vi "Draw Trajectory.vi"(0 "Picture in":refnum<vi>, 1 "Robot Index":i32, 5 "Trajectory Data":T3, 7 "time":dbl, 9 "new picture in":picture, 10 "MEGA?":bool, 11 "Hide Path":bool, 12 "MEGA traj":T2 {"?"."Limits"."StoopidFast (fps)" min=0.0; "?"."Limits"."Jerk (fps^3)" min=0.0 step=1.0; "?"."Limits"."Accel (fps^2)" min=0.0; "?"."Limits"."Velocity (fps)" min=0.0; "?"."Overrides"."Angle Override" step=5.0; "?"."Overrides"."Velocity Override" step=5.0; "?"."Overrides"."Angular Override" step=5.0; "?"."Angular Limits"."Jerk (deg/s^3)" min=0.0 step=1.0; "?"."Angular Limits"."Accel (deg/s^2)" min=0.0; "?"."Angular Limits"."Velocity (deg/s)" min=0.0}, 13 "color(black)":u32(colorbox)=6618880) -> (3 "Path Points MEGA":cluster{"x":dbl, "y":dbl}[][](array[cluster]), 4 "new picture":picture, 6 "Output Point":T12, 14 "Output Point MEGA":T1(array[cluster]), 15 "Path Points":cluster{"x":dbl, "y":dbl}[](array[cluster]))   [LabVIEW 2025]
uses:
  Types/Trajectory Data.ctl
  Types/Segment Type.ctl
  FileIO/MEGA traj.ctl
  Types/Single Cmd Info.ctl
  <vilib>/picture/picture.llb/imagedata.ctl
  Types/Limits.ctl
  Types/Overrides.ctl
  Types/Angluar Limits.ctl
  Types/Drive Type.ctl
  Types/Path Type.ctl
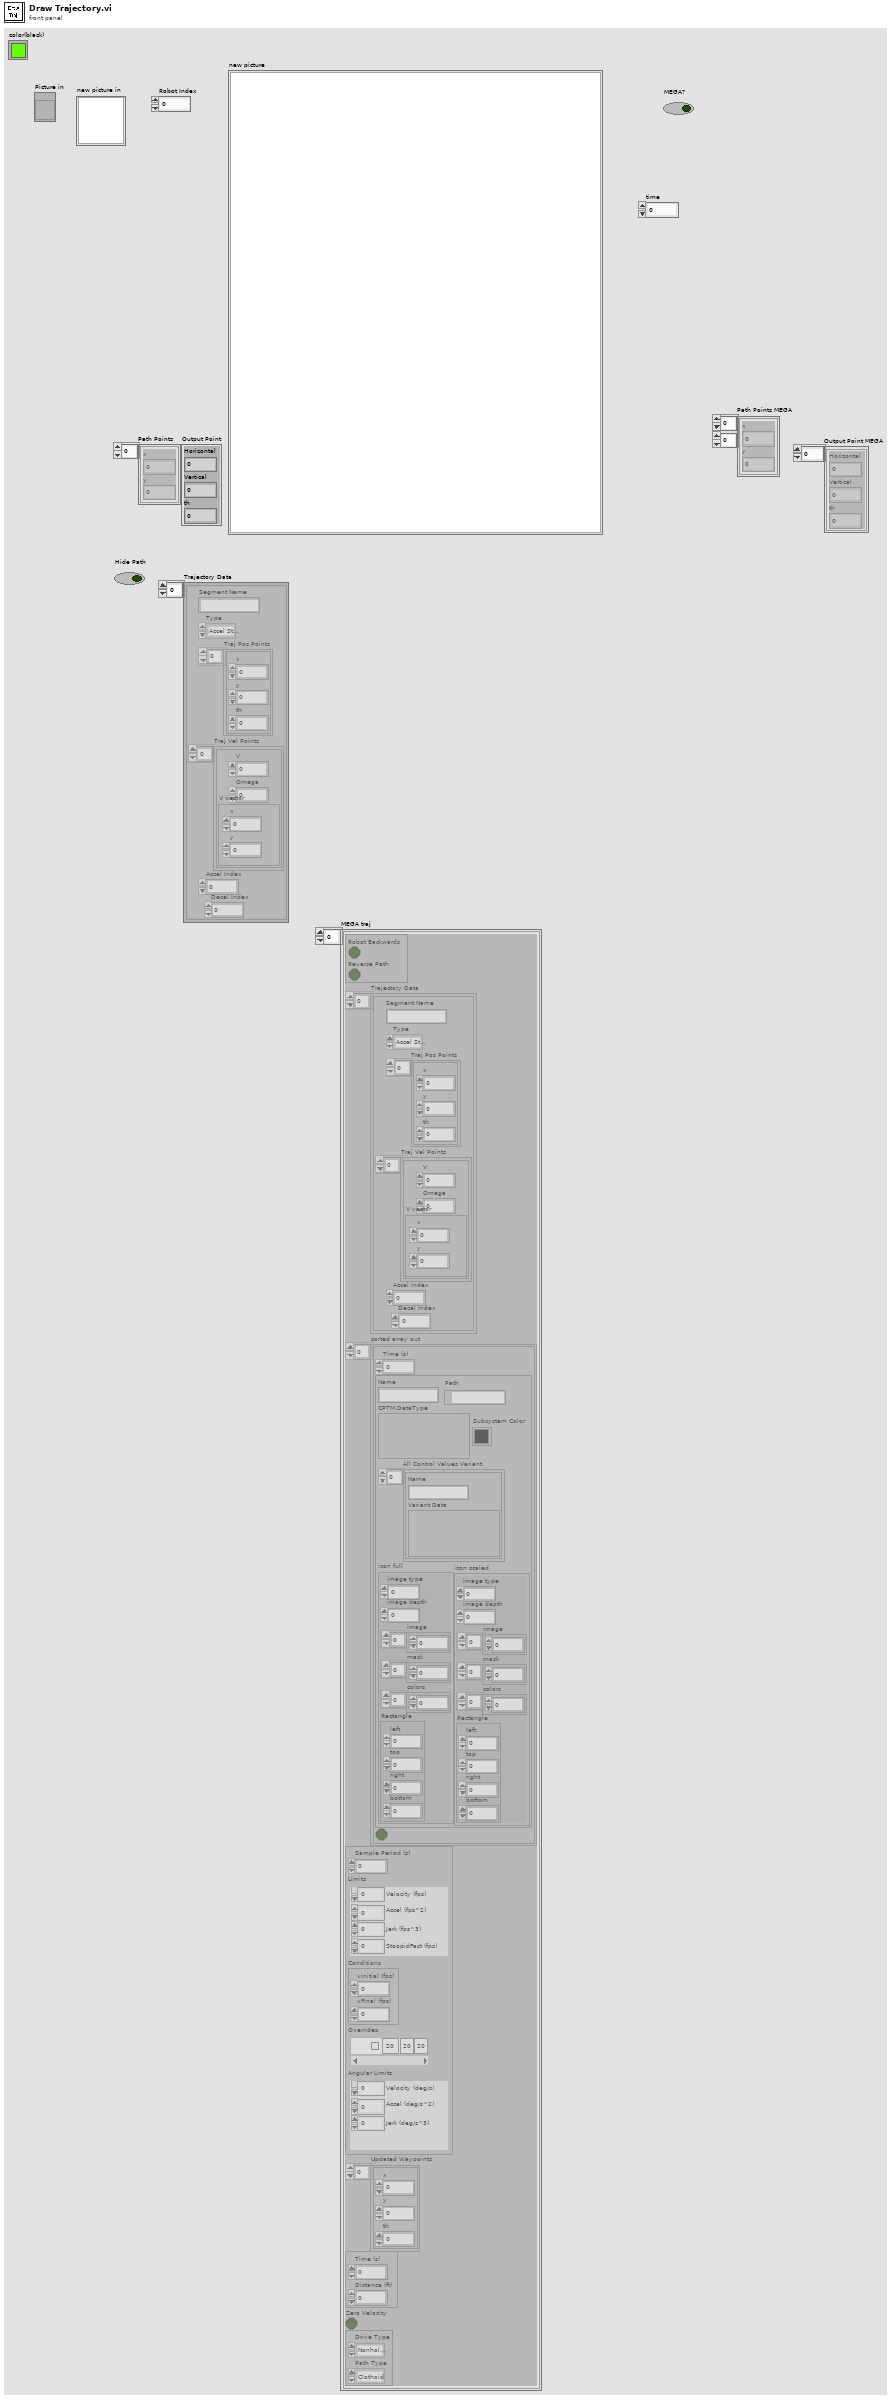
[diagram p1: front panel]
types:
  T1 = cluster{"Horizontal":dbl, "Vertical":dbl, "th":dbl}[]
  T2 = typedef "MEGA traj.ctl" = cluster{cluster{"Robot Backwards":bool, "Reverse Path":bool}, "Trajectory Data":T3, "sorted array out":cluster{"Time (s)":dbl, T5, bool}[], cluster{"Sample Period (s)":dbl, "Limits":T7, "Conditions":cluster{"vInitial (fps)":dbl, "vFinal (fps)":dbl}, "Overrides":T8, "Angular Limits":T9}, "Updated Waypoints":cluster{"x":dbl, "y":dbl, "th":dbl}[], cluster{"Time (s)":dbl, "Distance (ft)":dbl}, "Zero Velocity":bool, cluster{"Drive Type":T10, "Path Type":T11}}[]
  T3 = typedef "Trajectory Data.ctl" = cluster{"Segment Name":string, "Type":T4, "Traj Pos Points":cluster{"x":dbl, "y":dbl, "th":dbl}[], "Traj Vel Points":cluster{"V":dbl, "Omega":dbl, "V vector":cluster{"y":dbl, "x":dbl}}[], "Accel Index":i32, "Decel Index":i32}[]
  T4 = typedef "Segment Type.ctl" = enum16{"Accel Straight", "Const Straight", "Blend", "Circle", "Bezier"}
  T5 = typedef "Single Cmd Info.ctl" = cluster{"Name":string, "CPTM.DataType":variant, "All Control Values Variant":cluster{"Name":string, "Variant Data":variant}[], "icon full":T6, "icon scaled":T6, "Path":path, "Subsystem Color":u32}
  T6 = typedef "imagedata.ctl" = cluster{"image type":i32, "image depth":i32, "image":u8[], "mask":u8[], "colors":u32[], "Rectangle":cluster{"left":i16, "top":i16, "right":i16, "bottom":i16}}
  T7 = typedef "Limits.ctl" = cluster{"Velocity (fps)":dbl, "Accel (fps^2)":dbl, "Jerk (fps^3)":dbl, "StoopidFast (fps)":dbl}
  T8 = typedef "Overrides.ctl" = cluster{"Count":string, "Angular Override":dbl, "Enabled?":bool, "Velocity Override":dbl, "Angle Override":dbl}[]
  T9 = typedef "Angluar Limits.ctl" = cluster{"Velocity (deg/s)":dbl, "Accel (deg/s^2)":dbl, "Jerk (deg/s^3)":dbl}
  T10 = typedef "Drive Type.ctl" = enum16{"Nonholonomic", "Holonomic"}
  T11 = typedef "Path Type.ctl" = enum16{"Clothoid", "Bezier"}
  T12 = cluster{"Horizontal":dbl, "Vertical":dbl, "th":dbl}
  T13 = cluster{"Width":u16, "Style":enum32{"Solid", "Dash", "Dot", "DashDot", "DashDotDot"}}
  T14 = typedef "LVPositionTypeDef.ctl" = cluster{"Left":i32, "Top":i32}
  T15 = typedef "LVBoundsTypeDef.ctl" = cluster{"Width":u32, "Height":u32}
  T16 = cluster{"V":dbl, "Omega":dbl, "V vector":cluster{"y":dbl, "x":dbl}}[]
  T17 = cluster{cluster{"Robot Backwards":bool, "Reverse Path":bool}, "Trajectory Data":T3, "sorted array out":cluster{"Time (s)":dbl, T5, bool}[], cluster{"Sample Period (s)":dbl, "Limits":T7, "Conditions":cluster{"vInitial (fps)":dbl, "vFinal (fps)":dbl}, "Overrides":T8, "Angular Limits":T9}, "Updated Waypoints":cluster{"x":dbl, "y":dbl, "th":dbl}[], cluster{"Time (s)":dbl, "Distance (ft)":dbl}, "Zero Velocity":bool, cluster{"Drive Type":T10, "Path Type":T11}}
  T18 = cluster{"Robot Backwards":bool, "Reverse Path":bool}
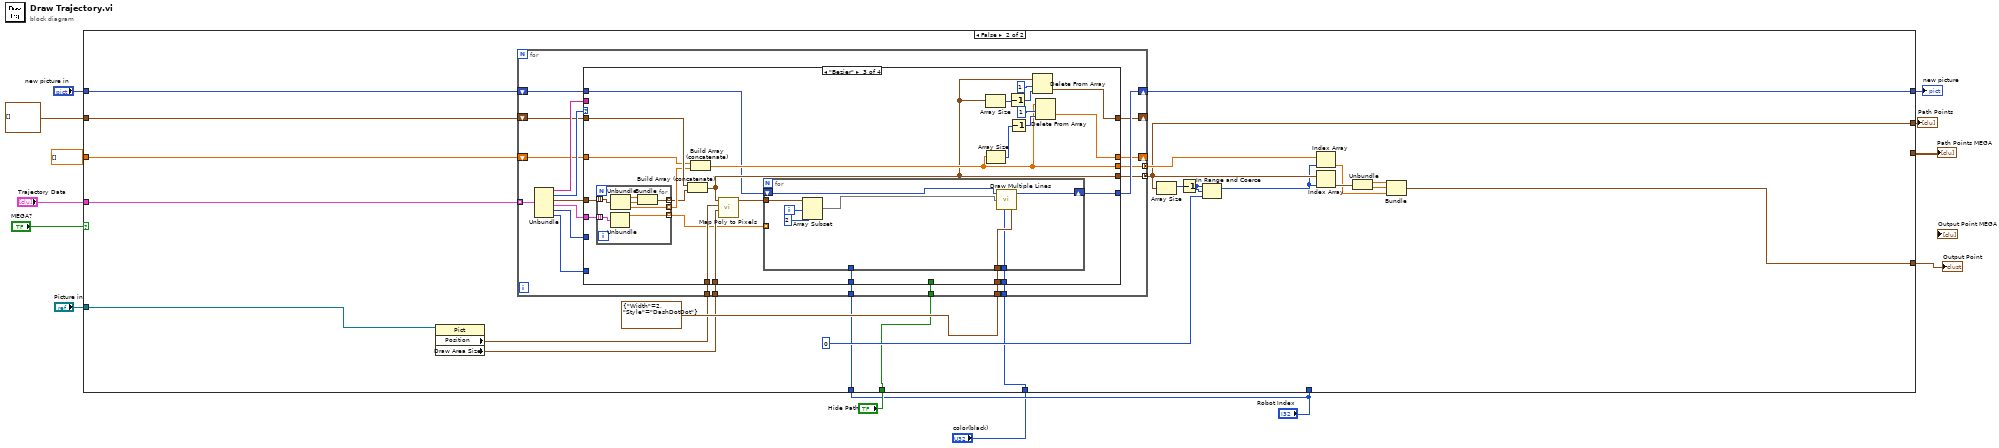
[diagram p0: block diagram]
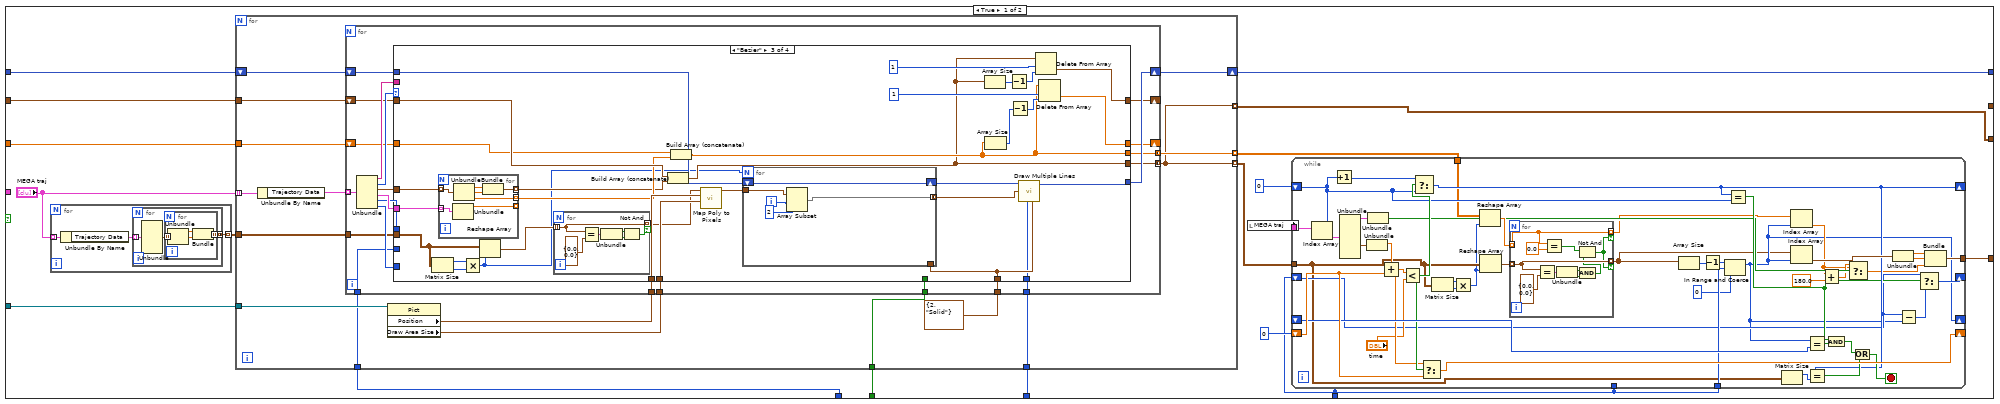
[diagram p2: hidden frame]
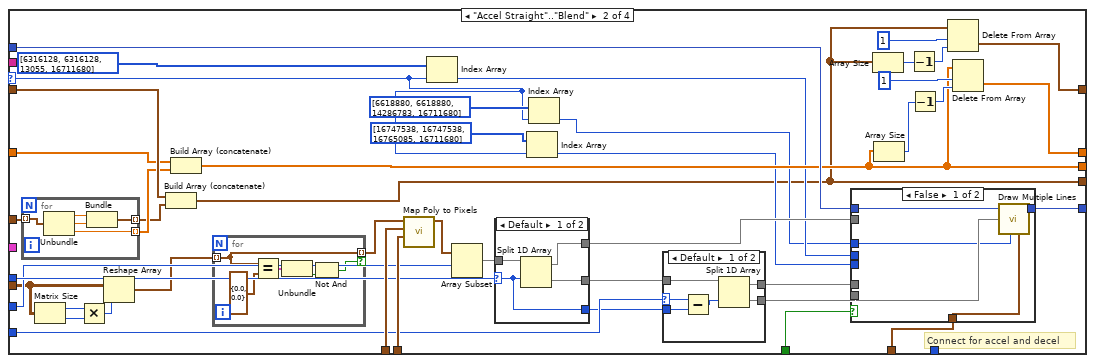
[diagram p4: hidden frame]
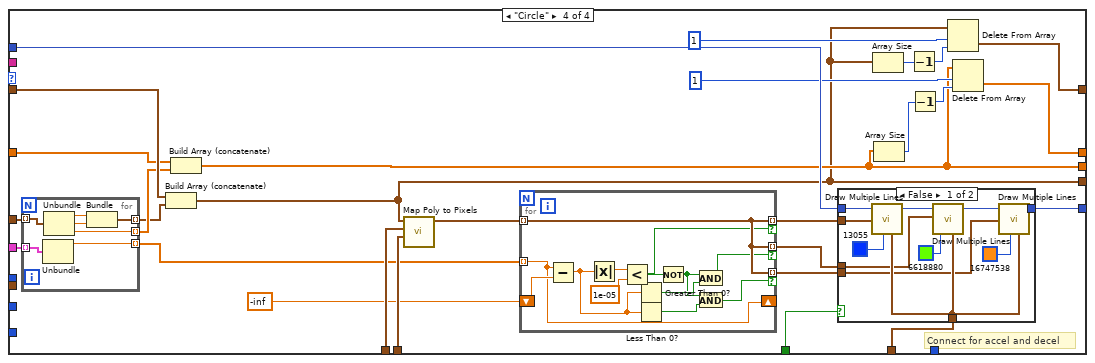
[diagram p8: hidden frame]
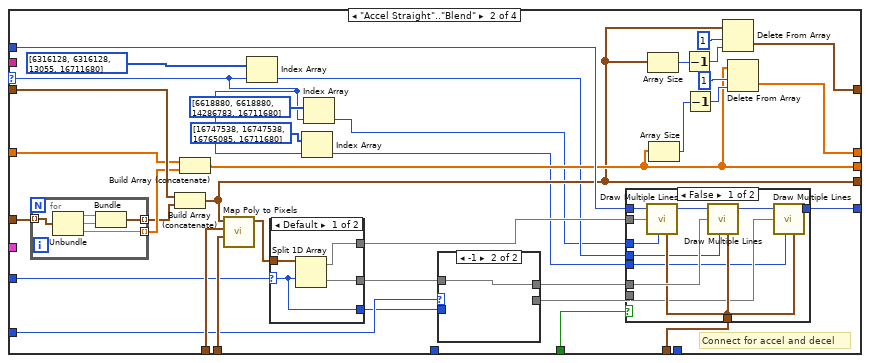
[diagram p11: hidden frame]
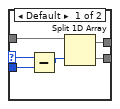
[diagram p13: hidden frame]
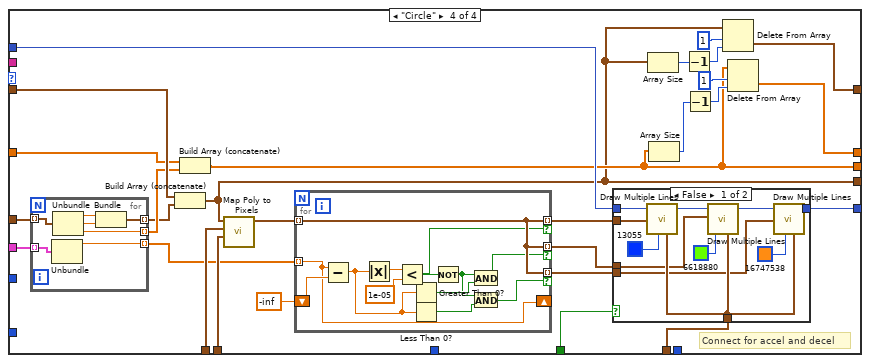
[diagram p15: hidden frame]
diagram:
  n1 = case shown="False" "MEGA?" {
    tunnel: "Picture in" -> [w31 w342]
    tunnel: "new picture in" -> [w30 w341]
    tunnel: [w29 w337] -> w11
    tunnel: [_ w331] -> w10
    tunnel: cluster{"x":dbl, "y":dbl}[] [] -> [w28 w327]
    tunnel: dbl[] [] -> [w27 w326]
    tunnel: "Trajectory Data" -> [_ w325]
    tunnel: "Hide Path" -> [w26 w324]
    tunnel: [w19 _] -> w4
    tunnel: "Robot Index" -> [w18 _]
    tunnel: [w23 w323] -> w3
    tunnel: "Robot Index" -> [w17 w322]
    tunnel: "color(black)" -> [w14 w321]
    frame True {
      n2 = for {
        tunnel: "MEGA traj" -> [w34] mode=indexing
        tunnel: [w32] -> w15 mode=indexing
        n3 = Unbundle By Name(w34) -> ("Trajectory Data"=w33:T3)
        n4 = for {
          tunnel: w33 -> [w37] mode=indexing
          tunnel: [w35] -> w32 mode=concatenating
          n5 = Unbundle(w37) -> ("Traj Pos Points"=w36:cluster{"x":dbl, "y":dbl, "th":dbl}[])  [unwired: 5 out]
          n6 = for {
            tunnel: w36 -> [w39] mode=indexing
            tunnel: [w38] -> w35 mode=indexing
            n7 = Unbundle(w39) -> ("x"=w41:dbl, "y"=w40:dbl)  [unwired: 1 out]
            n8 = Bundle("x"=w41, "y"=w40) -> (w38:cluster{"x":dbl, "y":dbl})  [unwired: 1 in]
          }
        }
      }
      n9 = for {
        tunnel: w31 -> [w113]
        tunnel: [w102] -> w19 mode=indexing
        tunnel: w28 -> [w107]
        tunnel: w27 -> [w106]
        shift-right: [w108] -> w29
        shift-left: w30 -> [w112]
        tunnel: w26 -> [w105]
        tunnel: "MEGA traj" -> [w100] mode=indexing
        tunnel: [w103] -> w20 mode=indexing
        tunnel: [w102] -> w21 mode=indexing
        tunnel: w17 -> [w101]
        tunnel: w15 -> [w99]
        tunnel: w14 -> [w98]
        n10 = Unbundle By Name(w100) -> ("Trajectory Data"=w104:T3)
        n11 = property on="Property Node" class="Pict"(reference=w113) -> ("Position"=w109:T14, "Draw Area Size"=w110:T15)  [unwired: 1 in, 2 out]
        n12 = for {
          tunnel: w104 -> [w135] mode=indexing
          shift-right: [w129] -> w108
          shift-left: w112 -> [w128]
          tunnel: T13 {"Width"=2, "Style"=enum."Solid"} ("pen") -> [w132]
          tunnel: w110 -> [w131]
          tunnel: w109 -> [w130]
          tunnel: [w126] -> w102 mode=concatenating
          tunnel: [w125] -> w103 mode=concatenating
          shift-right: [w124] -> _
          shift-left: w107 -> [w123]
          shift-right: [w122] -> _
          shift-left: w106 -> [w121]
          tunnel: w105 -> [w119]
          tunnel: w101 -> [w116]
          tunnel: w99 -> [w115]
          tunnel: w98 -> [w114]
          n13 = Unbundle(w135) -> ("Segment Name"=w134:string, "Type"=w127:T4, "Traj Pos Points"=w117:cluster{"x":dbl, "y":dbl, "th":dbl}[], "Traj Vel Points"=w133:T16, "Accel Index"=w118:i32, "Decel Index"=w120:i32)
          n14 = case shown="\"Bezier\"" w127 {
            selector: w127 -> [_ w152 _ _]
            tunnel: w134 -> [_ _ _ _]
            tunnel: w117 -> [_ w182 w242 w288]
            tunnel: w133 -> [_ _ w225 w267]
            tunnel: w132 -> [_ w161 w215 w271]
            tunnel: w131 -> [_ w181 w241 w287]
            tunnel: w130 -> [_ w179 w240 w285]
            tunnel: [w138 w162 w214 w272] -> w129
            tunnel: w128 -> [w138 w180 w224 w286]
            tunnel: [_ w146 w226 w269] -> w126
            tunnel: [_ w168 w230 w275] -> w125
            tunnel: w118 -> [_ w165 _ _]
            tunnel: [w137 w173 w235 w280] -> w124
            tunnel: w123 -> [w137 w176 w238 w283]
            tunnel: [w136 w169 w231 w276] -> w122
            tunnel: w121 -> [w136 w166 w228 w273]
            tunnel: w120 -> [_ w164 _ _]
            tunnel: w119 -> [_ w149 _ w268]
            tunnel: w116 -> [_ w145 _ _]
            tunnel: w115 -> [_ w144 w221 _]
            tunnel: w114 -> [_ _ w212 _]
            frame Default {
            }
            frame "Accel Straight".."Blend" {
              # "Connect for accel and decel"
              n15 = for {
                tunnel: w182 -> [w211] mode=indexing
                tunnel: [w210] -> w157 mode=indexing
                tunnel: [w207] -> w167 mode=indexing
                n16 = Unbundle(w211) -> ("x"=w209:dbl, "y"=w208:dbl, "th"=w207:dbl)
                n17 = Bundle("x"=w209, "y"=w208) -> (w210:cluster{"x":dbl, "y":dbl})  [unwired: 1 in]
              }
              n18 = Matrix Size(0:w144) -> (1:w143:i32, 2:w142:i32)
              n19 = Multiply(x=w143, y=w142) -> (x*y=w141:i32)
              n20 = Reshape Array(w144, w141) -> (w140:cluster{"x":dbl, "y":dbl}[])
              n21 = Build Array (concatenate)(w176, w157) -> (w146:cluster{"x":dbl, "y":dbl}[])
              n22 = Build Array (concatenate)(w166, w167) -> (w168:dbl[])
              n23 = for {
                tunnel: w140 -> [w188] mode=indexing
                tunnel: [w188] -> w139 mode=indexing if=w183
                n24 = Equal?(x=w188, y=cluster{"x":dbl, "y":dbl} {"x"=0.0, "y"=0.0}) -> (x = y?=w186:cluster{"x":bool, "y":bool})
                n25 = Unbundle(w186) -> ("x"=w184:bool, "y"=w185:bool)
                n26 = Not And(1:w185, 2:w184) -> (0:w183:bool)
              }
              n27 = call "Map Poly to Pixels.vi"("Draw Area Size"=w181, "Position"=w179, "Coords"=w139) -> ("Coords"=w147:cluster{"Horizontal":dbl, "Vertical":dbl}[])  [unwired: 8 in]
              n28 = Index Array(array=u32[] [6316128, 6316128, 13055, 16711680], index=w152) -> (element=w155:u32)
              n29 = Array Subset(array=w147, index=w145) -> (w148:cluster{"Horizontal":dbl, "Vertical":dbl}[])  [unwired: 1 in]
              n30 = case shown="Default" w165 {
                selector: w165 -> [w202 _]
                tunnel: w148 -> [w205 w206]
                tunnel: [w203 _] -> w156
                tunnel: [w204 w206] -> w159
                tunnel: [w202 _] -> w158
                frame Default {
                  n31 = Split 1D Array(array=w205, index=w202) -> (first subarray=w203:cluster{"Horizontal":dbl, "Vertical":dbl}[], second subarray=w204:cluster{"Horizontal":dbl, "Vertical":dbl}[])
                }
                frame -1 {
                }
              }
              n32 = Index Array(array=u32[] [16747538, 16747538, 16765085, 16711680], index=w152) -> (element=w150:u32)
              n33 = Index Array(array=u32[] [6618880, 6618880, 14286783, 16711680], index=w152) -> (element=w151:u32)
              n34 = case shown="Default" w164 {
                selector: w164 -> [w197 _]
                tunnel: w159 -> [w200 w201]
                tunnel: [w199 w201] -> w163
                tunnel: [w198 _] -> w160
                tunnel: w158 -> [w196 _]
                frame Default {
                  n35 = Subtract(x=w197, y=w196) -> (x-y=w195:i32)
                  n36 = Split 1D Array(array=w200, index=w195) -> (first subarray=w199:cluster{"Horizontal":dbl, "Vertical":dbl}[], second subarray=w198:cluster{"Horizontal":dbl, "Vertical":dbl}[])
                }
                frame -1 {
                }
              }
              n37 = case shown="False" w149 {
                tunnel: w180 -> [w190 w194]
                tunnel: w163 -> [_ _]
                tunnel: [w193 w194] -> w162
                tunnel: w161 -> [w192 _]
                tunnel: w160 -> [w191 _]
                tunnel: w156 -> [_ _]
                tunnel: w155 -> [_ _]
                tunnel: w151 -> [w189 _]
                tunnel: w150 -> [_ _]
                frame False {
                  n38 = call <vilib>:"Draw Multiple Lines.vi"("picture"=w190, "line endpoints"=w191, "color(black)"=w189, "pen"=w192) -> ("new picture"=w193:picture)  [unwired: 5 in]
                }
                frame True {
                }
              }
              n39 = Array Size(array=w146) -> (size(s)=w177:i32)
              n40 = Array Size(array=w168) -> (size(s)=w170:i32)
              n41 = Decrement(x=w177) -> (x-1=w174:i32)
              n42 = Decrement(x=w170) -> (x-1=w172:i32)
              n43 = Delete From Array(array=w146, length=1, index=w174) -> (deleted portion=w173:cluster{"x":dbl, "y":dbl}[])  [unwired: 1 out]
              n44 = Delete From Array(array=w168, length=1, index=w172) -> (deleted portion=w169:dbl[])  [unwired: 1 out]
            }
            frame "Bezier" {
              n45 = Matrix Size(0:w221) -> (1:w220:i32, 2:w223:i32)
              n46 = for {
                tunnel: w242 -> [w260] mode=indexing
                tunnel: [w259] -> w227 mode=indexing
                tunnel: [w256] -> w229 mode=indexing
                tunnel: w225 -> [w255] mode=indexing
                tunnel: [w254] -> _ mode=indexing
                n47 = Unbundle(w255) -> ("V"=w254:dbl)  [unwired: 2 out]
                n48 = Unbundle(w260) -> ("x"=w258:dbl, "y"=w257:dbl, "th"=w256:dbl)
                n49 = Bundle("x"=w258, "y"=w257) -> (w259:cluster{"x":dbl, "y":dbl})  [unwired: 1 in]
              }
              n50 = Multiply(x=w220, y=w223) -> (x*y=w213:i32)
              n51 = Reshape Array(w221, w213) -> (w222:cluster{"x":dbl, "y":dbl}[])
              n52 = for {
                tunnel: w222 -> [w248] mode=indexing
                tunnel: [w248] -> w219 mode=indexing if=w243
                n53 = Equal?(x=w248, y=cluster{"x":dbl, "y":dbl} {"x"=0.0, "y"=0.0}) -> (x = y?=w246:cluster{"x":bool, "y":bool})
                n54 = Unbundle(w246) -> ("x"=w244:bool, "y"=w245:bool)
                n55 = Not And(1:w245, 2:w244) -> (0:w243:bool)
              }
              n56 = Build Array (concatenate)(w238, w227) -> (w226:cluster{"x":dbl, "y":dbl}[])
              n57 = Build Array (concatenate)(w228, w229) -> (w230:dbl[])
              n58 = call "Map Poly to Pixels.vi"("Draw Area Size"=w241, "Position"=w240, "Coords"=w219) -> ("Coords"=w218:cluster{"Horizontal":dbl, "Vertical":dbl}[])  [unwired: 8 in]
              n59 = for {
                N: w213 -> [_]
                tunnel: w215 -> [_]
                shift-right: [w250] -> w217
                shift-left: w224 -> [w250]
                tunnel: w218 -> [w251]
                tunnel: [w249] -> w216 mode=concatenating
                i -> [w253]
                n60 = Array Subset(array=w251, index=w253, length=2) -> (w249:cluster{"Horizontal":dbl, "Vertical":dbl}[])
              }
              n61 = Array Size(array=w226) -> (size(s)=w239:i32)
              n62 = Array Size(array=w230) -> (size(s)=w232:i32)
              n63 = Decrement(x=w239) -> (x-1=w236:i32)
              n64 = Decrement(x=w232) -> (x-1=w234:i32)
              n65 = call <vilib>:"Draw Multiple Lines.vi"("picture"=w217, "line endpoints"=w216, "color(black)"=w212, "pen"=w215) -> ("new picture"=w214:picture)  [unwired: 5 in]
              n66 = Delete From Array(array=w226, length=1, index=w236) -> (deleted portion=w235:cluster{"x":dbl, "y":dbl}[])  [unwired: 1 out]
              n67 = Delete From Array(array=w230, length=1, index=w234) -> (deleted portion=w231:dbl[])  [unwired: 1 out]
            }
            frame "Circle" {
              # "Connect for accel and decel"
              n68 = for {
                tunnel: w288 -> [w319] mode=indexing
                tunnel: [w318] -> w270 mode=indexing
                tunnel: [w315] -> w274 mode=indexing
                tunnel: w267 -> [w314] mode=indexing
                tunnel: [w313] -> w266 mode=indexing
                n69 = Unbundle(w314) -> ("V"=w313:dbl)  [unwired: 2 out]
                n70 = Unbundle(w319) -> ("x"=w317:dbl, "y"=w316:dbl, "th"=w315:dbl)
                n71 = Bundle("x"=w317, "y"=w316) -> (w318:cluster{"x":dbl, "y":dbl})  [unwired: 1 in]
              }
              n72 = Build Array (concatenate)(w283, w270) -> (w269:cluster{"x":dbl, "y":dbl}[])
              n73 = Build Array (concatenate)(w273, w274) -> (w275:dbl[])
              n74 = call "Map Poly to Pixels.vi"("Draw Area Size"=w287, "Position"=w285, "Coords"=w269) -> ("Coords"=w261:cluster{"Horizontal":dbl, "Vertical":dbl}[])  [unwired: 8 in]
              n75 = for {
                tunnel: w261 -> [w297] mode=indexing
                tunnel: w266 -> [w296] mode=indexing
                shift-right: [w296] -> _
                shift-left: -inf -> [w300]
                tunnel: [w297] -> w264 mode=indexing if=w291
                tunnel: [w297] -> w263 mode=indexing if=w290
                tunnel: [w297] -> w262 mode=indexing if=w289
                n76 = Subtract(x=w296, y=w300) -> (x-y=w294:dbl)
                n77 = Absolute Value(x=w294) -> (abs(x)=w299:dbl)
                n78 = Less?(x=w299, y=1e-05) -> (x < y?=w291:bool)
                n79 = Greater Than 0?(x=w294) -> (x > 0?=w295:bool)
                n80 = Less Than 0?(x=w294) -> (x < 0?=w293:bool)
                n81 = Not(x=w291) -> (.not. x?=w292:bool)
                n82 = And(x=w292, y=w295) -> (x .and. y?=w290:bool)
                n83 = And(x=w292, y=w293) -> (x .and. y?=w289:bool)
              }
              n84 = case shown="False" w268 {
                tunnel: w286 -> [w311 w312]
                tunnel: [w308 w312] -> w272
                tunnel: w271 -> [w307 _]
                tunnel: w264 -> [w304 _]
                tunnel: w263 -> [w303 _]
                tunnel: w262 -> [w302 _]
                frame False {
                  n85 = call <vilib>:"Draw Multiple Lines.vi"("picture"=w311, "line endpoints"=w304, "color(black)"=u32 13055, "pen"=w307) -> ("new picture"=w310:picture)  [unwired: 5 in]
                  n86 = call <vilib>:"Draw Multiple Lines.vi"("picture"=w310, "line endpoints"=w303, "color(black)"=u32 6618880, "pen"=w307) -> ("new picture"=w309:picture)  [unwired: 5 in]
                  n87 = call <vilib>:"Draw Multiple Lines.vi"("picture"=w309, "line endpoints"=w302, "color(black)"=u32 16747538, "pen"=w307) -> ("new picture"=w308:picture)  [unwired: 5 in]
                }
                frame True {
                }
              }
              n88 = Array Size(array=w269) -> (size(s)=w284:i32)
              n89 = Array Size(array=w275) -> (size(s)=w277:i32)
              n90 = Decrement(x=w284) -> (x-1=w281:i32)
              n91 = Decrement(x=w277) -> (x-1=w279:i32)
              n92 = Delete From Array(array=w269, length=1, index=w281) -> (deleted portion=w280:cluster{"x":dbl, "y":dbl}[])  [unwired: 1 out]
              n93 = Delete From Array(array=w275, length=1, index=w279) -> (deleted portion=w276:dbl[])  [unwired: 1 out]
            }
          }
        }
      }
      n94 = local read "MEGA traj"() -> (w25:T2)
      n95 = while {
        tunnel: w18 -> [w63]
        tunnel: w21 -> [w58]
        tunnel: w20 -> [w59]
        shift-right: [w68] -> _
        shift-left: 0 -> [w67]
        tunnel: w25 -> [w86]
        shift-right: [w81] -> _
        shift-left: 0 -> [w82]
        shift-right: [w44] -> _
        shift-left: _ -> [w74]
        shift-right: [w66] -> _
        shift-left: w18 -> [w62]
        tunnel: [w52] -> w23
        tunnel: w18 -> [_]
        stop <- w75 stop-if-true
        n96 = Index Array(array=w86, index=w67) -> (element=w85:T17)
        n97 = Increment(x=w67) -> (x+1=w87:i32)
        n98 = Unbundle(w85) -> (w50:T18, w84:cluster{"Time (s)":dbl, "Distance (ft)":dbl})  [unwired: 6 out]
        n99 = Unbundle(w84) -> ("Time (s)"=w83:dbl)  [unwired: 1 out]
        n100 = Unbundle(w50) -> ("Robot Backwards"=w49:bool)  [unwired: 1 out]
        n101 = Add(x=w83, y=w82) -> (x+y=w72:dbl)
        n102 = Less?(x=w72, y="time") -> (x < y?=w73:bool)
        n103 = Select(t=w87, s=w73, f=w67) -> (s? t:f=w68:i32)
        n104 = Select(t=w72, s=w73, f=w82) -> (s? t:f=w81:dbl)
        n105 = Matrix Size(0:w58) -> (1:w57:i32, 2:w56:i32)
        n106 = Multiply(x=w57, y=w56) -> (x*y=w55:i32)
        n107 = Reshape Array(w59, w55) -> (w53:dbl[])
        n108 = Reshape Array(w58, w55) -> (w54:cluster{"x":dbl, "y":dbl}[])
        n109 = for {
          tunnel: w54 -> [w97] mode=indexing
          tunnel: [w97] -> w42 mode=indexing if=w90
          tunnel: w53 -> [w94] mode=indexing
          tunnel: [w94] -> w43 mode=indexing if=w90
          n110 = Equal?(x=w97, y=cluster{"x":dbl, "y":dbl} {"x"=0.0, "y"=0.0}) -> (x = y?=w95:cluster{"x":bool, "y":bool})
          n111 = Equal?(x=w94, y=0.0) -> (x = y?=w88:bool)
          n112 = Unbundle(w95) -> ("x"=w91:bool, "y"=w92:bool)
          n113 = And(x=w91, y=w92) -> (x .and. y?=w89:bool)
          n114 = Not And(1:w89, 2:w88) -> (0:w90:bool)
        }
        n115 = Array Size(array=w42) -> (size(s)=w60:i32)
        n116 = Decrement(x=w60) -> (x-1=w61:i32)
        n117 = In Range and Coerce(upper limit=w61, x=w63, lower limit=u16 0 ("Width")) -> (coerced(x)=w44:i32)  [unwired: 1 out]
        n118 = Equal?(x=w68, y=w67) -> (x = y?=w65:bool)
        n119 = Matrix Size(0:w58) -> (1:w77:i32)  [unwired: 1 out]
        n120 = Index Array(array=w43, index=w44) -> (element=w46:dbl)
        n121 = Index Array(array=w42, index=w44) -> (element=w80:cluster{"x":dbl, "y":dbl})
        n122 = Equal?(x=w44, y=w74) -> (x = y?=w70:bool)
        n123 = Equal?(x=w68, y=w77) -> (x = y?=w76:bool)
        n124 = Add(x=w46, y=180.0) -> (x+y=w47:dbl)
        n125 = And(x=w65, y=w70) -> (x .and. y?=w69:bool)
        n126 = Select(t=w47, s=w49, f=w46) -> (s? t:f=w48:dbl)
        n127 = Or(x=w69, y=w76) -> (x .or. y?=w75:bool)
        n128 = Unbundle(w80) -> ("x"=w79:dbl, "y"=w78:dbl)
        n129 = Subtract(x=w62, y=w44) -> (x-y=w64:i32)
        n130 = Select(t=w62, s=w65, f=w64) -> (s? t:f=w66:i32)
        n131 = Bundle("x"=w79, "y"=w78, "th"=w48) -> (w52:cluster{"x":dbl, "y":dbl, "th":dbl})  [unwired: 1 in]
      }
    }
    frame False {
      n132 = property on="Property Node" class="Pict"(reference=w342) -> ("Position"=w338:T14, "Draw Area Size"=w339:T15)  [unwired: 1 in, 2 out]
      n133 = for {
        tunnel: w325 -> [w363] mode=indexing
        shift-right: [w356] -> w337
        shift-left: w341 -> [w355]
        tunnel: T13 {"Width"=2, "Style"=enum."DashDotDot"} ("pen") -> [w359]
        tunnel: w339 -> [w358]
        tunnel: w338 -> [w357]
        tunnel: [w353] -> w331 mode=concatenating
        tunnel: [w352] -> w332 mode=concatenating
        shift-right: [w350] -> _
        shift-left: w327 -> [w349]
        shift-right: [w348] -> _
        shift-left: w326 -> [w347]
        tunnel: w324 -> [w345]
        tunnel: w322 -> [w344]
        tunnel: w321 -> [w343]
        n134 = Unbundle(w363) -> ("Segment Name"=w362:string, "Type"=w354:T4, "Traj Pos Points"=w361:cluster{"x":dbl, "y":dbl, "th":dbl}[], "Traj Vel Points"=w360:T16, "Accel Index"=w351:i32, "Decel Index"=w346:i32)
        n135 = case shown="\"Bezier\"" w354 {
          selector: w354 -> [_ w370 _ _]
          tunnel: w362 -> [_ _ _ _]
          tunnel: w361 -> [_ w402 w456 w499]
          tunnel: w360 -> [_ _ w439 w478]
          tunnel: w359 -> [_ w381 w434 w482]
          tunnel: w358 -> [_ w401 w455 w498]
          tunnel: w357 -> [_ w399 w454 w496]
          tunnel: [w366 w382 w435 w483] -> w356
          tunnel: w355 -> [w366 w400 w436 w497]
          tunnel: [_ w376 w440 w480] -> w353
          tunnel: [_ w388 w444 w486] -> w352
          tunnel: w351 -> [_ w385 _ _]
          tunnel: [w365 w393 w449 w491] -> w350
          tunnel: w349 -> [w365 w396 w452 w494]
          tunnel: [w364 w389 w445 w487] -> w348
          tunnel: w347 -> [w364 w386 w442 w484]
          tunnel: w346 -> [_ w384 _ _]
          tunnel: w345 -> [_ w367 _ w479]
          tunnel: w344 -> [_ _ w433 _]
          tunnel: w343 -> [_ _ w432 _]
          frame Default {
          }
          frame "Accel Straight".."Blend" {
            # "Connect for accel and decel"
            n136 = for {
              tunnel: w402 -> [w431] mode=indexing
              tunnel: [w430] -> w377 mode=indexing
              tunnel: [w427] -> w387 mode=indexing
              n137 = Unbundle(w431) -> ("x"=w429:dbl, "y"=w428:dbl, "th"=w427:dbl)
              n138 = Bundle("x"=w429, "y"=w428) -> (w430:cluster{"x":dbl, "y":dbl})  [unwired: 1 in]
            }
            n139 = Build Array (concatenate)(w396, w377) -> (w376:cluster{"x":dbl, "y":dbl}[])
            n140 = Build Array (concatenate)(w386, w387) -> (w388:dbl[])
            n141 = call "Map Poly to Pixels.vi"("Draw Area Size"=w401, "Position"=w399, "Coords"=w376) -> ("Coords"=w375:cluster{"Horizontal":dbl, "Vertical":dbl}[])  [unwired: 8 in]
            n142 = Index Array(array=u32[] [6316128, 6316128, 13055, 16711680], index=w370) -> (element=w373:u32)
            n143 = case shown="Default" w385 {
              selector: w385 -> [w422 _]
              tunnel: w375 -> [w425 w426]
              tunnel: [w423 _] -> w374
              tunnel: [w424 w426] -> w379
              tunnel: [w422 _] -> w378
              frame Default {
                n144 = Split 1D Array(array=w425, index=w422) -> (first subarray=w423:cluster{"Horizontal":dbl, "Vertical":dbl}[], second subarray=w424:cluster{"Horizontal":dbl, "Vertical":dbl}[])
              }
              frame -1 {
              }
            }
            n145 = Index Array(array=u32[] [16747538, 16747538, 16765085, 16711680], index=w370) -> (element=w368:u32)
            n146 = Index Array(array=u32[] [6618880, 6618880, 14286783, 16711680], index=w370) -> (element=w369:u32)
            n147 = case shown="-1" w384 {
              selector: w384 -> [w417 _]
              tunnel: w379 -> [w420 w421]
              tunnel: [w419 w421] -> w383
              tunnel: [w418 _] -> w380
              tunnel: w378 -> [w416 _]
              frame Default {
                n148 = Subtract(x=w417, y=w416) -> (x-y=w415:i32)
                n149 = Split 1D Array(array=w420, index=w415) -> (first subarray=w419:cluster{"Horizontal":dbl, "Vertical":dbl}[], second subarray=w418:cluster{"Horizontal":dbl, "Vertical":dbl}[])
              }
              frame -1 {
              }
            }
            n150 = case shown="False" w367 {
              tunnel: w400 -> [w413 w414]
              tunnel: w383 -> [w411 _]
              tunnel: [w409 w414] -> w382
              tunnel: w381 -> [w408 _]
              tunnel: w380 -> [w407 _]
              tunnel: w374 -> [w406 _]
              tunnel: w373 -> [w405 _]
              tunnel: w369 -> [w404 _]
              tunnel: w368 -> [w403 _]
              frame False {
                n151 = call <vilib>:"Draw Multiple Lines.vi"("picture"=w413, "line endpoints"=w406, "color(black)"=w404, "pen"=w408) -> ("new picture"=w412:picture)  [unwired: 5 in]
                n152 = call <vilib>:"Draw Multiple Lines.vi"("picture"=w412, "line endpoints"=w411, "color(black)"=w405, "pen"=w408) -> ("new picture"=w410:picture)  [unwired: 5 in]
                n153 = call <vilib>:"Draw Multiple Lines.vi"("picture"=w410, "line endpoints"=w407, "color(black)"=w403, "pen"=w408) -> ("new picture"=w409:picture)  [unwired: 5 in]
              }
              frame True {
              }
            }
            n154 = Array Size(array=w376) -> (size(s)=w397:i32)
            n155 = Array Size(array=w388) -> (size(s)=w390:i32)
            n156 = Decrement(x=w397) -> (x-1=w394:i32)
            n157 = Decrement(x=w390) -> (x-1=w392:i32)
            n158 = Delete From Array(array=w376, length=1, index=w394) -> (deleted portion=w393:cluster{"x":dbl, "y":dbl}[])  [unwired: 1 out]
            n159 = Delete From Array(array=w388, length=1, index=w392) -> (deleted portion=w389:dbl[])  [unwired: 1 out]
          }
          frame "Bezier" {
            n160 = for {
              tunnel: w456 -> [w471] mode=indexing
              tunnel: [w470] -> w441 mode=indexing
              tunnel: [w467] -> w443 mode=indexing
              tunnel: w439 -> [w466] mode=indexing
              tunnel: [w465] -> w438 mode=indexing
              n161 = Unbundle(w466) -> ("V"=w465:dbl)  [unwired: 2 out]
              n162 = Unbundle(w471) -> ("x"=w469:dbl, "y"=w468:dbl, "th"=w467:dbl)
              n163 = Bundle("x"=w469, "y"=w468) -> (w470:cluster{"x":dbl, "y":dbl})  [unwired: 1 in]
            }
            n164 = Build Array (concatenate)(w452, w441) -> (w440:cluster{"x":dbl, "y":dbl}[])
            n165 = Build Array (concatenate)(w442, w443) -> (w444:dbl[])
            n166 = call "Map Poly to Pixels.vi"("Draw Area Size"=w455, "Position"=w454, "Coords"=w440) -> ("Coords"=w437:cluster{"Horizontal":dbl, "Vertical":dbl}[])  [unwired: 8 in]
            n167 = for {
              tunnel: w437 -> [w461]
              tunnel: w434 -> [w464]
              shift-right: [w458] -> w435
              shift-left: w436 -> [w463]
              tunnel: w433 -> [_]
              tunnel: w438 -> [_] mode=indexing
              tunnel: w432 -> [w457]
              i -> [w460]
              n168 = Array Subset(array=w461, index=w460, length=2) -> (w459:cluster{"Horizontal":dbl, "Vertical":dbl}[])
              n169 = call <vilib>:"Draw Multiple Lines.vi"("picture"=w463, "line endpoints"=w459, "color(black)"=w457, "pen"=w464) -> ("new picture"=w458:picture)  [unwired: 5 in]
            }
            n170 = Array Size(array=w440) -> (size(s)=w453:i32)
            n171 = Array Size(array=w444) -> (size(s)=w446:i32)
            n172 = Decrement(x=w453) -> (x-1=w450:i32)
            n173 = Decrement(x=w446) -> (x-1=w448:i32)
            n174 = Delete From Array(array=w440, length=1, index=w450) -> (deleted portion=w449:cluster{"x":dbl, "y":dbl}[])  [unwired: 1 out]
            n175 = Delete From Array(array=w444, length=1, index=w448) -> (deleted portion=w445:dbl[])  [unwired: 1 out]
          }
          frame "Circle" {
            # "Connect for accel and decel"
            n176 = for {
              tunnel: w499 -> [w530] mode=indexing
              tunnel: [w529] -> w481 mode=indexing
              tunnel: [w526] -> w485 mode=indexing
              tunnel: w478 -> [w525] mode=indexing
              tunnel: [w524] -> w476 mode=indexing
              n177 = Unbundle(w525) -> ("V"=w524:dbl)  [unwired: 2 out]
              n178 = Unbundle(w530) -> ("x"=w528:dbl, "y"=w527:dbl, "th"=w526:dbl)
              n179 = Bundle("x"=w528, "y"=w527) -> (w529:cluster{"x":dbl, "y":dbl})  [unwired: 1 in]
            }
            n180 = Build Array (concatenate)(w494, w481) -> (w480:cluster{"x":dbl, "y":dbl}[])
            n181 = Build Array (concatenate)(w484, w485) -> (w486:dbl[])
            n182 = call "Map Poly to Pixels.vi"("Draw Area Size"=w498, "Position"=w496, "Coords"=w480) -> ("Coords"=w477:cluster{"Horizontal":dbl, "Vertical":dbl}[])  [unwired: 8 in]
            n183 = for {
              tunnel: w477 -> [w508] mode=indexing
              tunnel: w476 -> [w507] mode=indexing
              shift-right: [w507] -> _
              shift-left: -inf -> [w511]
              tunnel: [w508] -> w474 mode=indexing if=w502
              tunnel: [w508] -> w473 mode=indexing if=w501
              tunnel: [w508] -> w472 mode=indexing if=w500
              n184 = Subtract(x=w507, y=w511) -> (x-y=w505:dbl)
              n185 = Absolute Value(x=w505) -> (abs(x)=w510:dbl)
              n186 = Less?(x=w510, y=1e-05) -> (x < y?=w502:bool)
              n187 = Greater Than 0?(x=w505) -> (x > 0?=w506:bool)
              n188 = Less Than 0?(x=w505) -> (x < 0?=w504:bool)
              n189 = Not(x=w502) -> (.not. x?=w503:bool)
              n190 = And(x=w503, y=w506) -> (x .and. y?=w501:bool)
              n191 = And(x=w503, y=w504) -> (x .and. y?=w500:bool)
            }
            n192 = case shown="False" w479 {
              tunnel: w497 -> [w522 w523]
              tunnel: [w519 w523] -> w483
              tunnel: w482 -> [w518 _]
              tunnel: w474 -> [w515 _]
              tunnel: w473 -> [w514 _]
              tunnel: w472 -> [w513 _]
              frame False {
                n193 = call <vilib>:"Draw Multiple Lines.vi"("picture"=w522, "line endpoints"=w515, "color(black)"=u32 13055, "pen"=w518) -> ("new picture"=w521:picture)  [unwired: 5 in]
                n194 = call <vilib>:"Draw Multiple Lines.vi"("picture"=w521, "line endpoints"=w514, "color(black)"=u32 6618880, "pen"=w518) -> ("new picture"=w520:picture)  [unwired: 5 in]
                n195 = call <vilib>:"Draw Multiple Lines.vi"("picture"=w520, "line endpoints"=w513, "color(black)"=u32 16747538, "pen"=w518) -> ("new picture"=w519:picture)  [unwired: 5 in]
              }
              frame True {
              }
            }
            n196 = Array Size(array=w480) -> (size(s)=w495:i32)
            n197 = Array Size(array=w486) -> (size(s)=w488:i32)
            n198 = Decrement(x=w495) -> (x-1=w492:i32)
            n199 = Decrement(x=w488) -> (x-1=w490:i32)
            n200 = Delete From Array(array=w480, length=1, index=w492) -> (deleted portion=w491:cluster{"x":dbl, "y":dbl}[])  [unwired: 1 out]
            n201 = Delete From Array(array=w486, length=1, index=w490) -> (deleted portion=w487:dbl[])  [unwired: 1 out]
          }
        }
      }
      n202 = Array Size(array=w331) -> (size(s)=w330:i32)
      n203 = Decrement(x=w330) -> (x-1=w320:i32)
      n204 = In Range and Coerce(upper limit=w320, x=w320, lower limit=u16 0 ("Width")) -> (coerced(x)=w328:i32)  [unwired: 1 out]
      n205 = Index Array(array=w332, index=w328) -> (element=w333:dbl)
      n206 = Index Array(array=w331, index=w328) -> (element=w336:cluster{"x":dbl, "y":dbl})
      n207 = Unbundle(w336) -> ("x"=w335:dbl, "y"=w334:dbl)
      n208 = Bundle("x"=w335, "y"=w334, "th"=w333) -> (w323:cluster{"x":dbl, "y":dbl, "th":dbl})  [unwired: 1 in]
    }
  }
  "new picture" <- w11
  "Path Points" <- w10
  "Path Points MEGA" <- w4
  "Output Point" <- w3
